vi "DODividerConfig.vi"(0 "object in":refnum<class "AD2_DO_SDK.lvclass">, 2 "DOSingleCh":T1 {"IdleState" items=["PushPull", "OpenDrain", "OpenSource", "TriState"]; "DigitalOutOutput" items=["Pulse", "Custom", "Random"]; "Type" items=["Pulse", "Custom", "Random"]}, 5 "error in (no error)":errorcluster) -> (14 "object out":refnum<class "AD2_DO_SDK.lvclass">, 16 "DOSingleCh Out":T1 {"IdleState" items=["PushPull", "OpenDrain", "OpenSource", "TriState"]; "DigitalOutOutput" items=["Pulse", "Custom", "Random"]; "Type" items=["Pulse", "Custom", "Random"]}, 19 "error out":errorcluster)   [LabVIEW 2021, in "AD2_DO_SDK.lvclass"]
uses:
  AD2_DO_SDK.lvclass
  DOSingleCh.ctl
  AD2_DO_SDK.lvclass/AD2_DO_SDK.ctl
  Olasdwf/Olasdwf.lvlib
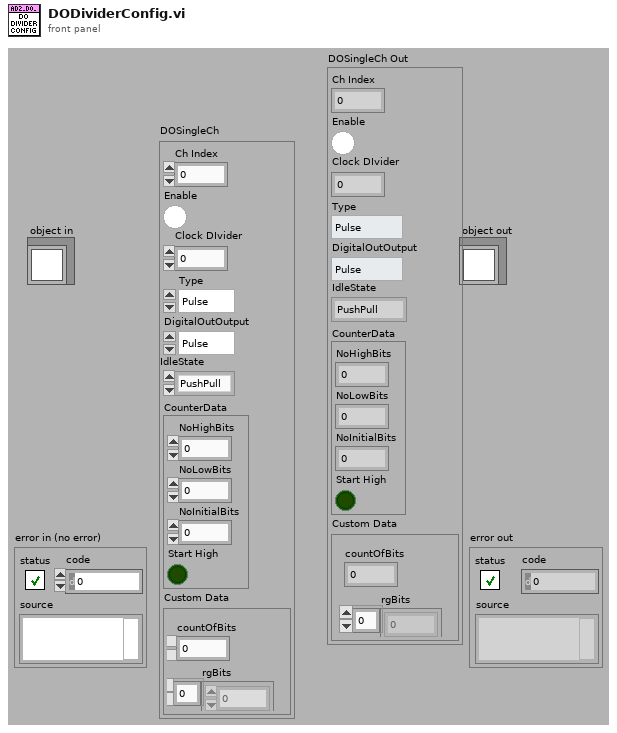
[diagram p1: front panel]
types:
  T1 = typedef "AD2_DO_SDK.lvclass/DOSingleCh.ctl" = cluster{"Ch Index":i32, "Enable":bool, "Clock DIvider":u32, "Type":i32, "DigitalOutOutput":u16, "IdleState":u16, "CounterData":cluster{"NoHighBits":u32, "NoLowBits":u32, "NoInitialBits":u32, "Start High":bool}, "Custom Data":cluster{"countOfBits":u32, "rgBits":u8[]}}
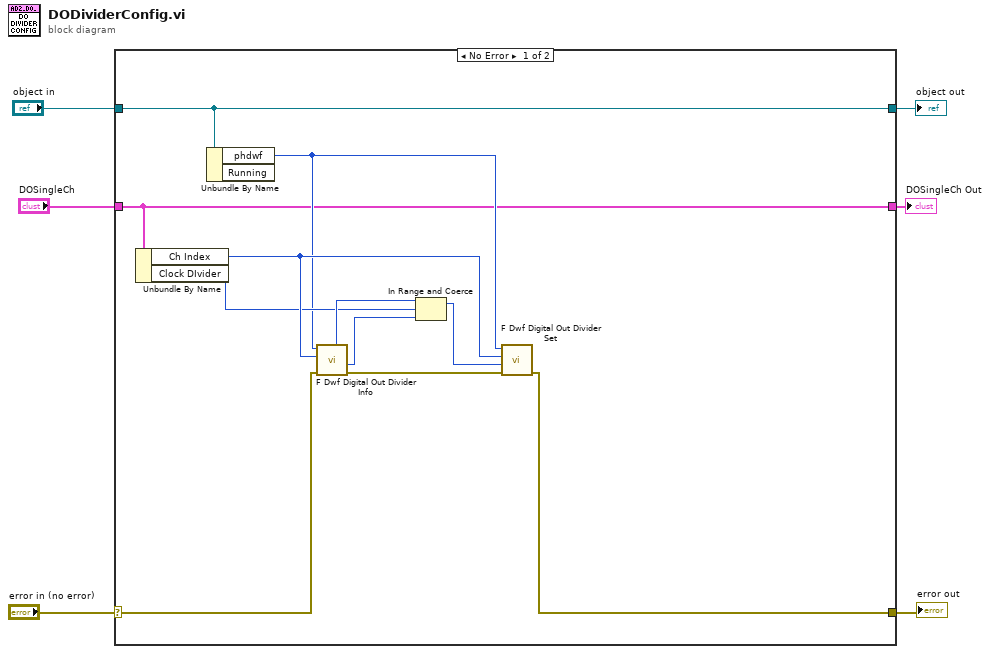
[diagram p0: block diagram]
diagram:
  n1 = case shown="No Error" "error in (no error)" {
    selector: "error in (no error)" -> [w10 w20]
    tunnel: [w7 w20] -> w5
    tunnel: [w11 w19] -> w3
    tunnel: "object in" -> [w11 w19]
    tunnel: "DOSingleCh" -> [w8 w18]
    tunnel: [w8 w18] -> w1
    frame No Error {
      n2 = Unbundle By Name(w8) -> ("Ch Index"=w14:i32, "Clock DIvider"=w13:u32)
      n3 = Unbundle By Name(w11) -> ("phdwf"=w9:i32)  [unwired: 1 out]
      n4 = call "F Dwf Digital Out Divider Info.vi"("error in (no error)"=w10, "idxChannel"=w14, "hdwf"=w9) -> ("error out"=w15:errorcluster, "vMin out"=w17:u32, "vMax out"=w16:u32)  [unwired: 5 in, 1 out]
      n5 = In Range and Coerce(upper limit=w16, x=w13, lower limit=w17) -> (coerced(x)=w12:u32)  [unwired: 1 out]
      n6 = call "F Dwf Digital Out Divider Set.vi"("error in (no error)"=w15, "v"=w12, "idxChannel"=w14, "hdwf"=w9) -> ("error out"=w7:errorcluster)  [unwired: 6 in, 1 out]
    }
    frame Error {
    }
  }
  "error out" <- w5
  "object out" <- w3
  "DOSingleCh Out" <- w1
